vi "Parse Remote Terminal.vi"(8 "error in (no error)":errorcluster, 11 "Single RT XML Node":refnum<k20>) -> (0 "error out":errorcluster, 3 "Single RT":refnum<class "Remote Terminal.lvclass">[](array[class]))   [LabVIEW 2020]
doc: "Retrieves all the Remote Terminals defined for a single bus in XML."
uses:
  Remote Terminal/Remote Terminal.lvclass
  Remote Terminal/TypeDefs/RT Configuration.ctl
  Remote Terminal/TypeDefs/RT-RT Timeout.ctl
  Remote Terminal/TypeDefs/Mode Code 17 Sync Configuration.ctl
  Remote Terminal/TypeDefs/RT Timetag Configuration.ctl
  Remote Terminal/TypeDefs/RT Command Config.ctl
  Frames & Messages/TypeDefs/Command Type.ctl
  Frames & Messages/TypeDefs/Command SubAddress.ctl
  Frames & Messages/TypeDefs/Command Word Count.ctl
  Frames & Messages/TypeDefs/Simplified Parameter Data Table.ctl
  Frames & Messages/TypeDefs/Scaling Information.ctl
  <vilib>/xml/NI_XML.lvlib
  BCI-1553 API.lvlib
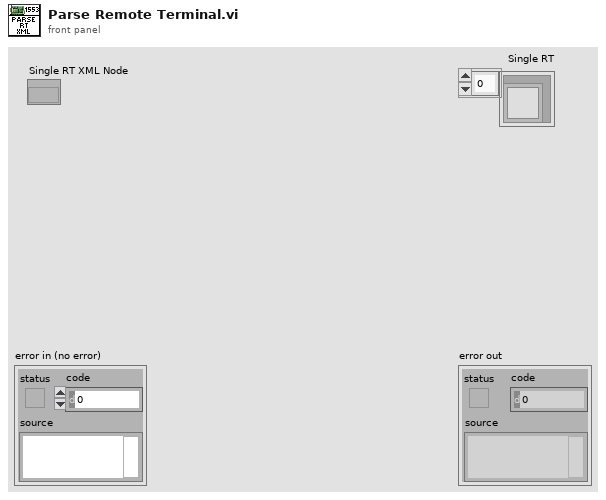
[diagram p1: front panel]
types:
  T1 = typedef "BCI-1553 API.lvlib/Remote Terminal.lvclass/RT Configuration.ctl" = cluster{"RT-RT Timeout":T2, "Inhibit Bus A":bool, "Inhibit Bus B":bool, "Broadcast CMD Invalid":bool, "UnDef MCs Invalid":bool, "Notice 2 Data Storage":bool, "SMCP":bool, "Temp RX Buffer":bool, "Alt BIT Enable":bool, "Auto Bus Shutdown":bool, "MC 16 SR Reset":bool, "MC 17 Sync":T3, "MC 8 Reset":bool, "Remote Terminal Timetag Config":T4}
  T2 = typedef "BCI-1553 API.lvlib/Remote Terminal.lvclass/RT-RT Timeout.ctl" = enum16{"57us", "62us", "100us", "180us"}
  T3 = typedef "BCI-1553 API.lvlib/Remote Terminal.lvclass/Mode Code 17 Sync Configuration.ctl" = enum16{"Sync if Bit 0 = 1", "Sync if Bit 0 = 0", "Sync Unconditionally"}
  T4 = typedef "BCI-1553 API.lvlib/Remote Terminal.lvclass/RT Timetag Configuration.ctl" = enum16{"Disabled", "2us", "4us", "8us", "16us", "32us", "64us"}
  T5 = typedef "BCI-1553 API.lvlib/Remote Terminal.lvclass/RT Command Config.ctl" = cluster{"Command Type":T6, "SubAddress":T7, "Word Count\\Mode Code":T8, "Initial Data":u16[], "Data Fields":T9[]}
  T6 = typedef "BCI-1553 API.lvlib/Command Type.ctl" = enum16{"Transmit", "Receive"}
  T7 = typedef "BCI-1553 API.lvlib/Command SubAddress.ctl" = enum16{"Mode Code", "1", "2", "3", "4", "5", "6", "7", "8", "9", "10", "11", "12", "13", "14", "15", "16", "17", "18", "19", "20", "21", "22", "23", "24", "25", "26", "27", "28", "29", "30"}
  T8 = typedef "BCI-1553 API.lvlib/Command Word Count.ctl" = enum16{"1", "2", "3", "4", "5", "6", "7", "8", "9", "10", "11", "12", "13", "14", "15", "16", "17", "18", "19", "20", "21", "22", "23", "24", "25", "26", "27", "28", "29", "30", "31", "32"}
  T9 = typedef "BCI-1553 API.lvlib/Simplified Parameter Data Table.ctl" = cluster{"Parameter Name":string, "Base Word":u16, "Scaling Info":T10}
  T10 = typedef "BCI-1553 API.lvlib/Scaling Information.ctl" = cluster{"Bit Offset":i32, "Bit Count":i32, "LSB Resolution":dbl, "2's Complement":bool, "Big Endian":bool, "Sign Bit":bool}
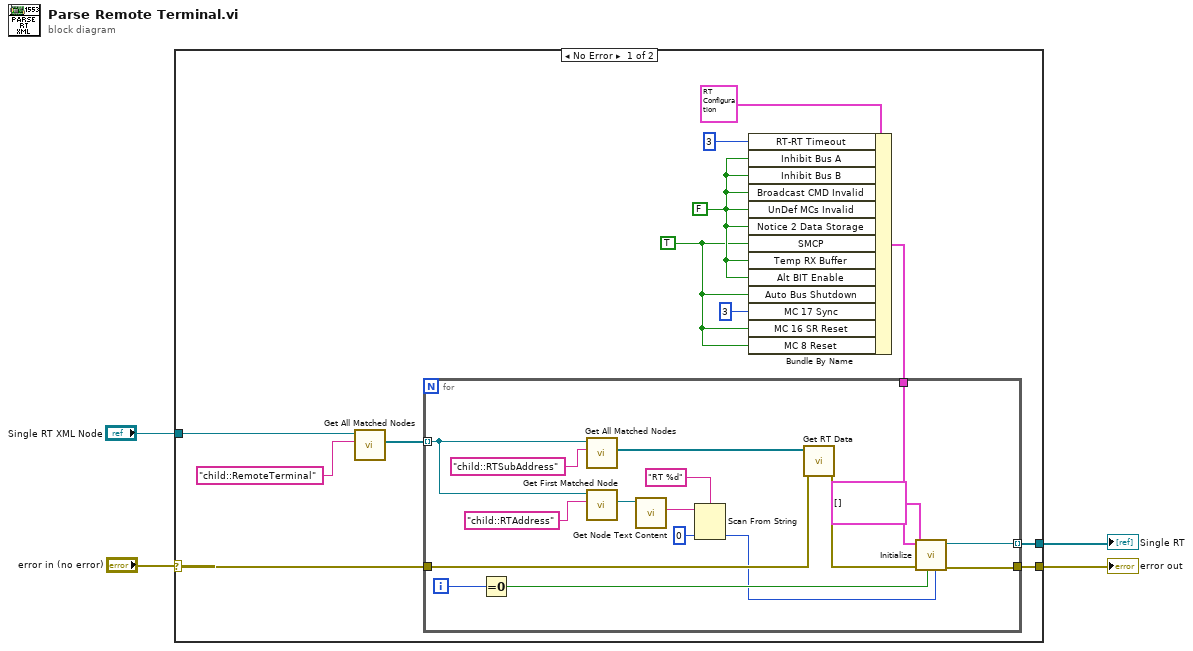
[diagram p0: block diagram]
diagram:
  n1 = case shown="No Error" "error in (no error)" {
    selector: "error in (no error)" -> [w6 w34]
    tunnel: [w16 w34] -> w3
    tunnel: "Single RT XML Node" -> [w14 _]
    tunnel: [w15 _] -> w1
    frame No Error {
      w7 = TRUE ("SMCP")
      w9 = FALSE ("UnDef MCs Invalid")
      n2 = call <vilib>:"Get All Matched Nodes.vi"("XPath expression"="child::RemoteTerminal", "node in"=w14) -> ("node result array"=w5:refnum<k20>[])  [unwired: 7 in, 2 out]
      n3 = Bundle By Name(cluster=T1 {"RT-RT Timeout"=enum."57us", "Inhibit Bus A"=FALSE, "Inhibit Bus B"=FALSE, "Broadcast CMD Invalid"=FALSE, "UnDef MCs Invalid"=FALSE, "Notice 2 Data Storage"=FALSE, "SMCP"=FALSE, "Temp RX Buffer"=FALSE, "Alt BIT Enable"=FALSE, "Auto Bus Shutdown"=FALSE, "MC 16 SR Reset"=FALSE, "MC 17 Sync"=enum."Sync if Bit 0 = 1", "MC 8 Reset"=FALSE, "Remote Terminal Timetag Config"=enum."Disabled"} ("RT Configuration"), "RT-RT Timeout"=u8 3 ("RT-RT TimeOut (us)"), "Inhibit Bus A"=w9, "Inhibit Bus B"=w9, "Broadcast CMD Invalid"=w9, "UnDef MCs Invalid"=w9, "Notice 2 Data Storage"=w9, "SMCP"=w7, "Temp RX Buffer"=w9, "Alt BIT Enable"=w9, "Auto Bus Shutdown"=w7, "MC 17 Sync"=u8 3, "MC 16 SR Reset"=w7, "MC 8 Reset"=w7) -> (w11:T1)
      n4 = for {
        tunnel: [w27] -> w15 mode=indexing
        tunnel: w11 -> [w32]
        tunnel: w6 -> [w29]
        tunnel: [w33] -> w16
        tunnel: w5 -> [w25] mode=indexing
        i -> [w23]
        n5 = Equal To 0?(x=w23) -> (x = 0?=w22:bool)
        n6 = call <vilib>:"Get All Matched Nodes.vi"("XPath expression"="child::RTSubAddress", "node in"=w25) -> ("node result array"=w30:refnum<k20>[])  [unwired: 7 in, 2 out]
        n7 = call <vilib>:"Get First Matched Node.vi"("XPath expression"="child::RTAddress", "node in"=w25) -> ("node result"=w24:refnum<k20>)  [unwired: 7 in, 2 out]
        n8 = call <vilib>:"Get Node Text Content.vi"("node in"=w24) -> ("node text"=w21:string)  [unwired: 8 in, 2 out]
        n9 = Scan From String(format string="RT %d", input string=w21, default 1=u8 0 ("default value 1")) -> (output 1=w19:u8)  [unwired: 2 in, 3 out]
        n10 = call "Get RT Data.vi"("error in (no error)"=w29, "RT SubAddresses XML Ref"=w30) -> ("error out"=w28:errorcluster)  [unwired: 8 in, 1 out]
        n11 = call "Initialize.vi"("Terminal Address"=w19, "RT 1?"=w22, "error in (no error)"=w28, "RT Commands"=T5[] [], "RT Configuration"=w32) -> ("error out"=w33:errorcluster, "Remote Terminal out"=w27:refnum<class "Remote Terminal.lvclass">)  [unwired: 5 in]
      }
    }
    frame Error {
    }
  }
  "error out" <- w3
  "Single RT" <- w1
